vi "Reserve Sessions.vi"(6 "timeout_in_milliseconds":i32, 8 "error in":errorcluster, 9 "Instrument Type Id":string, 10 "pin or relay names":string[](array[string]), 11 "Measurement Context In":refnum<class "MeasurementContext.lvclass">) -> (0 "error out":errorcluster, 1 "gRPC Device Location":T1, 2 "session information":T2[](array[typedef]), 3 "Measurement Context Out":refnum<class "MeasurementContext.lvclass">)   [LabVIEW 2020, in "MeasurementLink Measurement Server.lvlib"]
uses:
  MeasurementLink Measurement Server.lvlib
  Classes/MeasurementContext/MeasurementContext.lvclass
  <vilib>/MeasurementLink/MeasurementLink Session Management Client/RPC Messages/ni_measurementlink_sessionmanagement_v1_SessionInformation.ctl
  <vilib>/MeasurementLink/MeasurementLink Session Management Client/RPC Messages/nidevice_grpc_Session.ctl
  <vilib>/MeasurementLink/MeasurementLink Session Management Client/RPC Messages/ni_measurementlink_sessionmanagement_v1_ChannelMapping.ctl
  MeasurementLink Discovery Client/RPC Messages/ni_measurementlink_discovery_v1_ServiceLocation.ctl
  MeasurementLink Discovery Client/RPC Messages/ni_measurementlink_discovery_v1_ResolveServiceRequest.ctl
  <vilib>/MeasurementLink/MeasurementLink Session Management Client/RPC Messages/ni_measurementlink_sessionmanagement_v1_ReserveSessionsRequest.ctl
  <vilib>/MeasurementLink/MeasurementLink Session Management Client/RPC Messages/ni_measurementlink_PinMapContext.ctl
  Classes/MeasurementContext/MeasurementContext.lvclass/MeasurementContext.ctl
  Classes/MeasurementContext/Accessor/Write Session manager service gRPC ID.vi
  Classes/MeasurementContext/Accessor/Write Discovery service gRPC ID.vi
  MeasurementLink Discovery Client/MeasurementLink Discovery Client.lvlib
  <vilib>/MeasurementLink/MeasurementLink Session Management Client/MeasurementLink Session Management Client.lvlib
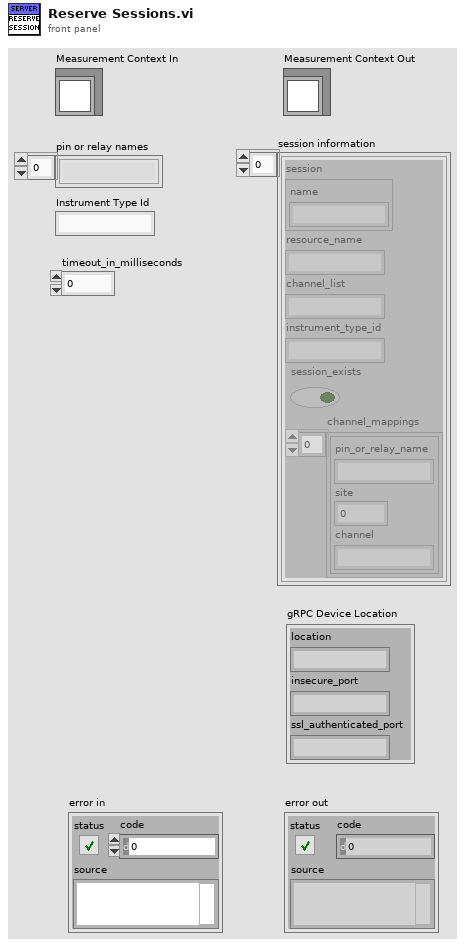
[diagram p1: front panel]
types:
  T1 = typedef "MeasurementLink Discovery Client.lvlib/ni_measurementlink_discovery_v1_ServiceLocation.ctl" = cluster{"location":string, "insecure_port":string, "ssl_authenticated_port":string}
  T2 = typedef "MeasurementLink Session Management Client.lvlib/ni_measurementlink_sessionmanagement_v1_SessionInformation.ctl" = cluster{"session":T3, "resource_name":string, "channel_list":string, "instrument_type_id":string, "session_exists":bool, "channel_mappings":T4[]}
  T3 = typedef "MeasurementLink Session Management Client.lvlib/nidevice_grpc_Session.ctl" = cluster{"name":string}
  T4 = typedef "MeasurementLink Session Management Client.lvlib/ni_measurementlink_sessionmanagement_v1_ChannelMapping.ctl" = cluster{"pin_or_relay_name":string, "site":i32, "channel":string}
  T5 = typedef "MeasurementLink Session Management Client.lvlib/ni_measurementlink_sessionmanagement_v1_ReserveSessionsRequest.ctl" = cluster{"pin_map_context":T6, "pin_or_relay_names":string[], "instrument_type_id":string, "timeout_in_milliseconds":i32}
  T6 = typedef "MeasurementLink Session Management Client.lvlib/ni_measurementlink_PinMapContext.ctl" = cluster{"pin_map_id":string, "sites":i32[]}
  T7 = typedef "MeasurementLink Discovery Client.lvlib/ni_measurementlink_discovery_v1_ResolveServiceRequest.ctl" = cluster{"provided_interface":string, "service_class":string}
  T8 = typedef "MeasurementLink Measurement Server.lvlib/PinMapContext.ctl" = cluster{"pin_map_id":string, "sites":i32[]}
  T9 = typedef "grpc-lvsupport-release.lvlib/grpcId.ctl" = u64
  T10 = typedef "MeasurementLink Session Management Client.lvlib/ni_measurementlink_sessionmanagement_v1_ReserveSessionsResponse.ctl" = cluster{"sessions":T2[]}
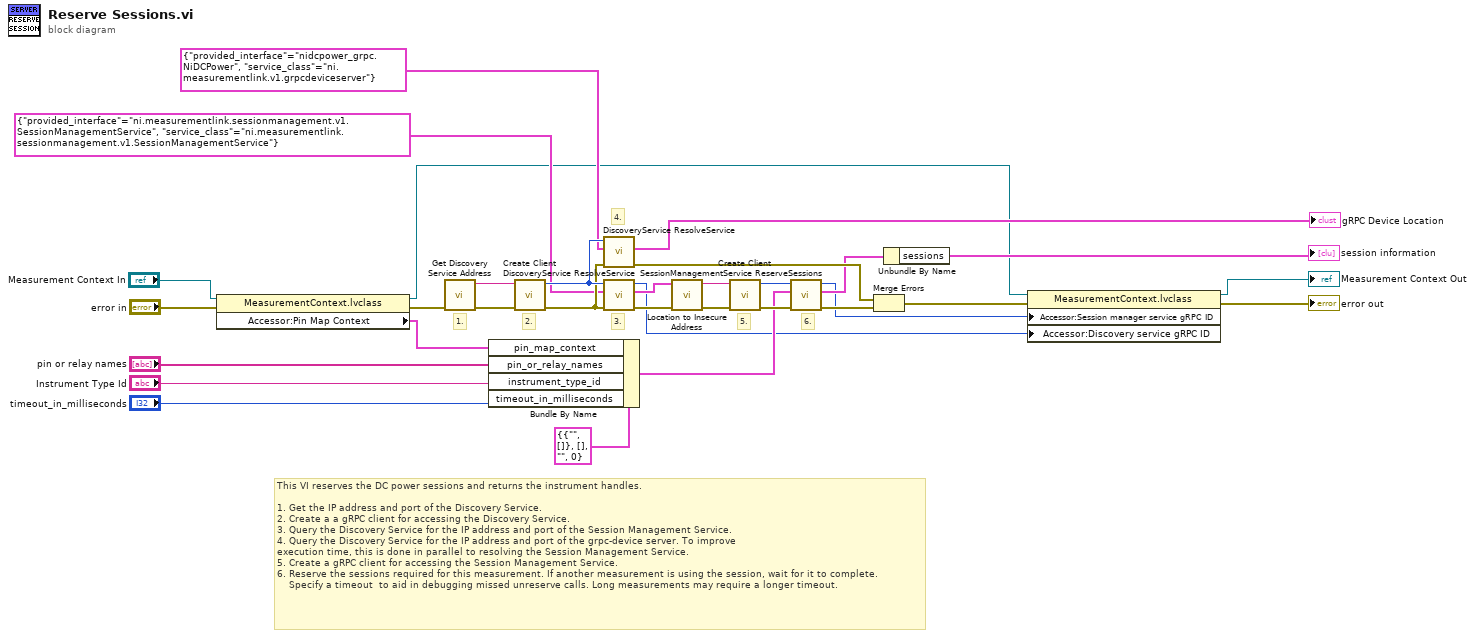
[diagram p0: block diagram]
diagram:
  # "6."
  # "5."
  # "4."
  # "3."
  # "2."
  # "1."
  # "This VI reserves the DC power sessions and returns the instrument handles.\n\n1. Get the IP address and port of the Discovery Service.\n2. Create a a gRPC client for accessing the Discovery Service.\n3. Query the Discovery Service for the IP address and port of the Session Management Service.\n4. Query the Discovery Service for the IP address and port of the grpc-device server. To improve \nexecution time, this is done in parallel to resolving the Session Management Service.\n5. Create a gRPC client for accessing the Session Management Service.\n6. Reserve the sessions required for this measurement. If another measurement is using the session, wait for it to complete. \n    Specify a timeout  to aid in debugging missed unreserve calls. Long measurements may require a longer timeout."
  n1 = property class="MeasurementContext.lvclass"(reference="Measurement Context In", error in="error in") -> (reference out=w4:refnum<class "MeasurementContext.lvclass">, error out=w12:errorcluster, "Accessor:Pin Map Context"=w10:T8)
  n2 = call "Get Discovery Service Address.vi"("error in"=w12) -> ("error out"=w31:errorcluster, "address"=w30:string)  [unwired: 9 in]
  n3 = Bundle By Name(cluster=T5 {"pin_map_context"={"pin_map_id"="", "sites"=[]}, "pin_or_relay_names"=[], "instrument_type_id"="", "timeout_in_milliseconds"=0} ("Request Data"), "pin_map_context"=w10, "pin_or_relay_names"="pin or relay names", "instrument_type_id"="Instrument Type Id", "timeout_in_milliseconds"="timeout_in_milliseconds") -> (w9:T5)
  n4 = call <vilib>:"Create Client.vi"("error in"=w31, "address"=w30) -> ("error out"=w21:errorcluster, "gRPC ID Out"=w22:T9)  [unwired: 8 in]
  n5 = call "DiscoveryService ResolveService.vi"("error in"=w21, "Request Data"=T7 {"provided_interface"="nidcpower_grpc.NiDCPower", "service_class"="ni.measurementlink.v1.grpcdeviceserver"}, "gRPC ID"=w22) -> ("error out"=w24:errorcluster, "Response Data"=→"gRPC Device Location":T1)  [unwired: 6 in, 1 out]
  n6 = call "DiscoveryService ResolveService.vi"("error in"=w21, "Request Data"=T7 {"provided_interface"="ni.measurementlink.sessionmanagement.v1.SessionManagementService", "service_class"="ni.measurementlink.sessionmanagement.v1.SessionManagementService"}, "gRPC ID"=w22) -> ("error out"=w25:errorcluster, "Response Data"=w29:T1, "gRPC ID out"=w2:T9)  [unwired: 6 in]
  n7 = call "Location to Insecure Address.vi"("Response Data"=w29) -> ("String"=w28:string)  [unwired: 10 in]
  n8 = call <vilib>:"Create Client.vi"("error in"=w25, "address"=w28) -> ("error out"=w26:errorcluster, "gRPC ID Out"=w27:T9)  [unwired: 8 in]
  n9 = call <vilib>:"SessionManagementService ReserveSessions.vi"("error in"=w26, "Request Data"=w9, "gRPC ID"=w27) -> ("error out"=w23:errorcluster, "Response Data"=w18:T10, "gRPC ID out"=w3:T9)  [unwired: 6 in]
  n10 = Merge Errors(w24, w23) -> (w17:errorcluster)
  n11 = Unbundle By Name(w18) -> ("sessions"=→"session information":T2[])
  n12 = property class="MeasurementContext.lvclass"(reference=w4, error in=w17, "Accessor:Session manager service gRPC ID"=w3, "Accessor:Discovery service gRPC ID"=w2) -> (reference out=→"Measurement Context Out":refnum<class "MeasurementContext.lvclass">, error out=→"error out":errorcluster)
